vi "Ratchet Brake.vi"(4 "Untension Speed":dbl=-0.1, 5 "Slow Extend":dbl=0.25, 6 "Brake Delay":dbl=0.2, 7 "Extend Speed":dbl=1.0, 8 "Reverse Time":dbl=0.4, 9 "Slow Retract":dbl=-0.25, 10 "Servo Disengage":i32, 11 "Retract Speed":dbl=-0.9, 12 "Retract":bool, 13 "Extend":bool, 14 "Slow":bool, 15 "Servo Engage":i32=120) -> (1 "Motor":dbl, 2 "Brake Servo":i32, 3 "State":enum16{"Engaged", "Untension", "Disengaged"}(ring))   [LabVIEW 2012]
panel:
  in  "Retract 2":bool
  in  "Extend 2":bool
  in  "Slow 2":bool
  out "State 2":enum16{"Engaged", "Untension", "Disengaged"}(ring)
  # "INPUTS"
  # "BRAKE SETTINGS"
  # "OUTPUTS"
  # "Disabled Code Implementation Example"
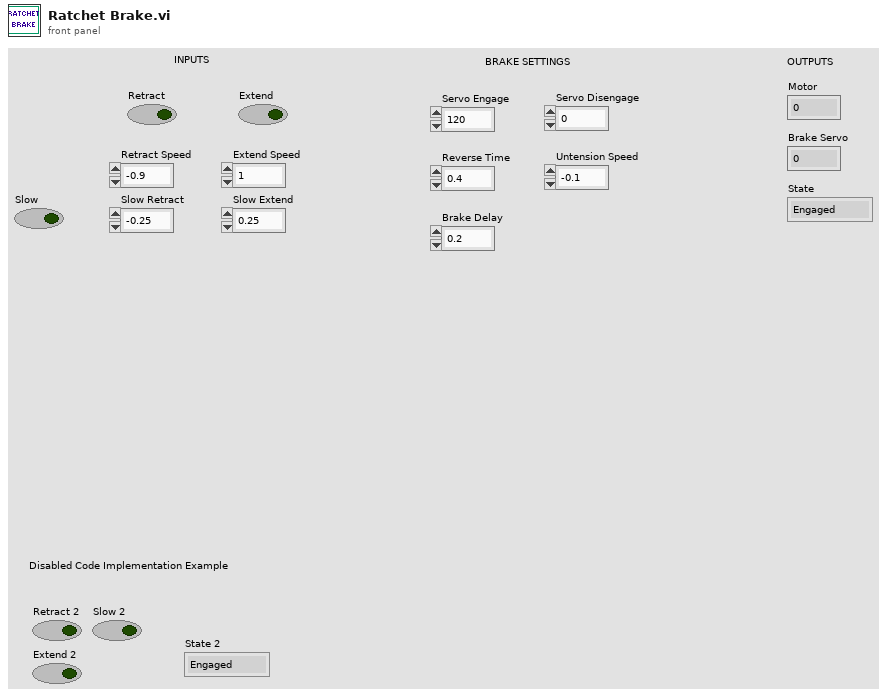
[diagram p1: front panel]
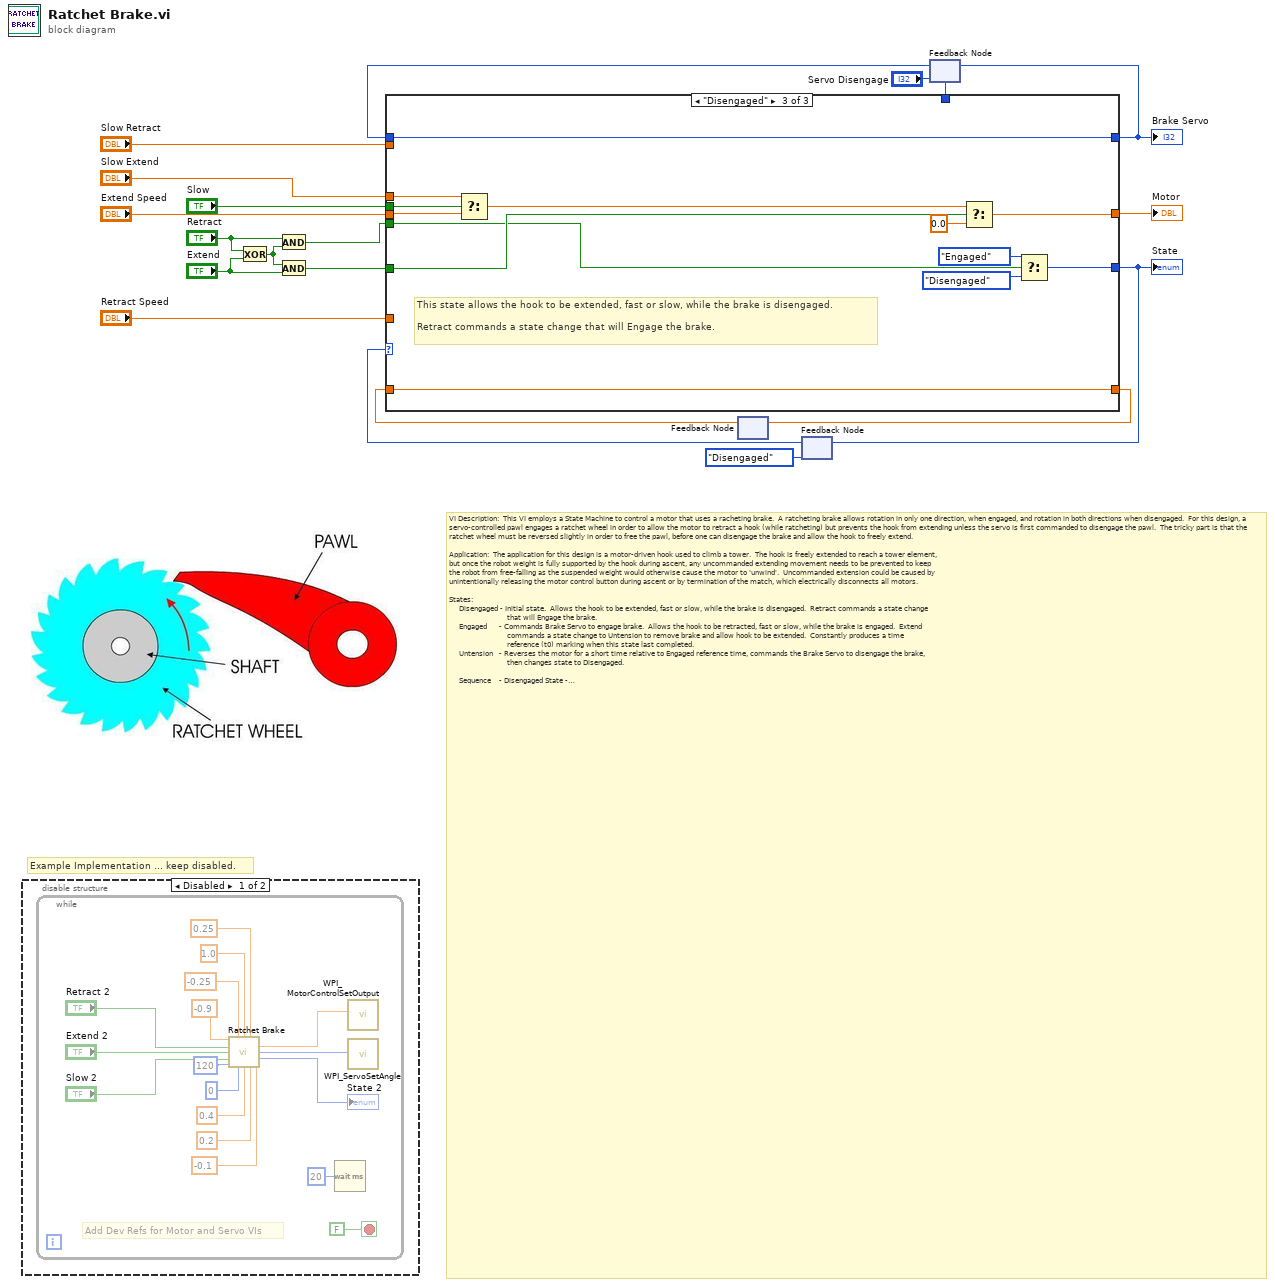
[diagram p0: block diagram]
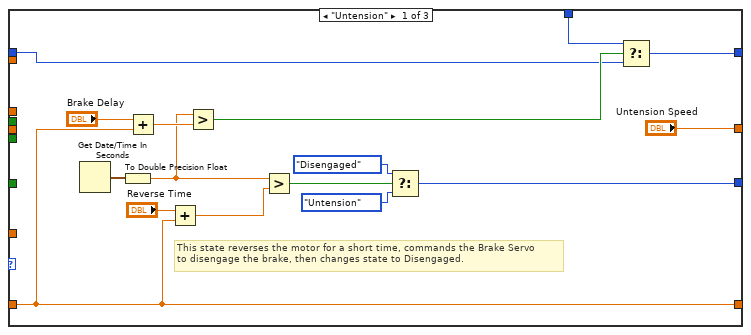
[diagram p3: hidden frame]
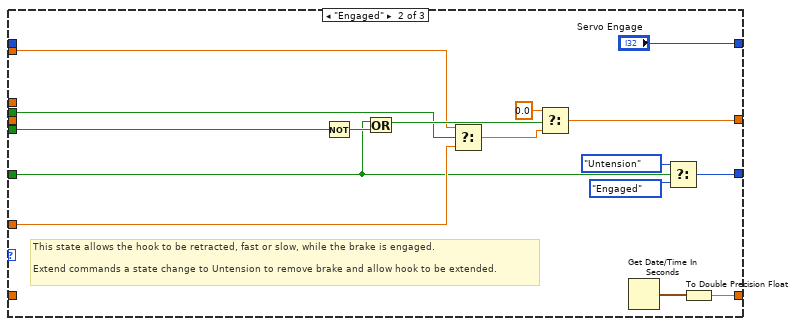
[diagram p4: hidden frame]
diagram:
  # "Example Implementation ... keep disabled."
  # "VI Description:  This VI employs a State Machine to control a motor that uses a racheting brake.  A ratcheting brake allows rotation in only one direction, when engaged, and rotation in both directions when disengaged.  For this design, a servo-controlled pawl engages a ratchet wheel in order to allow the motor to retract a hook (while ratcheting) but prevents the hook from extending unless the servo is first commanded to disengage the pawl.  The tricky part is that the ratchet wheel must be reversed slightly in order to free the pawl, before one can disengage the brake and allow the hook to freely extend.\n\nApplication:  The application for this design is a motor-driven hook used to climb a tower.  The hook is freely extended to reach a tower element,\nbut once the robot weight is fully supported by the hook during ascent, any uncommanded extending movement needs to be prevented to keep\nthe robot from free-falling as the suspended weight would otherwise cause the motor to 'unwind'.  Uncommanded extension could be caused by \nunintentionally releasing the motor control button during ascent or by termination of the match, which electrically disconnects all motors.\n\nStates:  \n     Disengaged - Initial state.  Allows the hook to be extended, fast or slow, while the brake is disengaged.  Retract commands a state change\n                             that will Engage the brake.\n     Engaged      - Commands Brake Servo to engage brake.  Allows the hook to be retracted, fast or slow, while the brake is engaged.  Extend \n                             commands a state change to Untension to remove brake and allow hook to be extended.  Constantly produces a time\n                             reference (t0) marking when this state last completed.\n     Untension   - Reverses the motor for a short time relative to Engaged reference time, commands the Brake Servo to disengage the brake,\n                             then changes state to Disengaged.\n\n     Sequence    - Disengaged State -> (on retract) -> Engaged State -> (on extend) -> Untension State -> Disengaged State\n\nThe state machine principle is that the brake is engaged whenever retracting (climbing).  The brake is untensioned by reversing the ratchet\nwheel upon an extend command.  This effectively allows extension to only occur when specifically commanded.\n\nInputs:\n     Extend                   - Boolean command to extend hook.  Simultaneous selection of Extend and Retract is considered ambigious and results in no change.\n     Retract                  - Boolean command to retract hook.  Simultaneous selection of Extend and Retract is considered ambigious and results in no change.\n     Slow                      - Use Slow Extend or Slow Retract motor values when True.\n     Extend Speed       - Motor value for fast extend.\n     Retract Speed      - Motor value for fast retract.\n     Slow Extend         - Motor value for slow extend.\n     Slow Retract         - Motor value for slow retract.\n     Untension Speed - Motor value to reverse motor while untensioning brake.\n     Reverse Time       - Time in seconds to reverse motor while untensioning brake.\n     Brake Delay          - Time in seconds to delay prior to commanding brake servo to remove brake pawl.\n     Servo Engage       - Servo position to move brake pawl into ratchet wheel.\n     Servo Disengage - Servo position to remove brake pawl from ratchet wheel.\n\nOutputs:\n     Brake Servo          - Current Brake Servo position.\n     Motor                   - Motor value output determined by state machine.\n     State                     - Current state of state machine.\n\nImplementation:\n     Determine Brake Servo positions for moving brake pawl into and out of ratchet wheel, and set Servo Engage and Disengage.\n     Determine a motor Untension Speed and Reverse Time combination that allows the brake pawl to be freed from the ratchet wheel at Brake\n           Delay seconds.  Reverse Time and Brake Delay will likely be fractions of a second, with Reverse Time >= Brake Delay.\n     Set Extend, Retract, and Slow speed motor values.  Extend and Retract will have opposite signs.  Untension Speed will have the same sign as Retract.\n\n\n----- RoboBees Team 836! -----  Control your freewheeling, think about a career in STEM! ..."
  n1 = disable-structure shown="Disabled" {
    frame Disabled {
      n2 = while {
        stop <- FALSE stop-if-true
        # "Add Dev Refs for Motor and Servo VIs"
        n3 = call "Ratchet Brake.vi"("Untension Speed"=-0.1, "Slow Extend"=0.25, "Brake Delay"=0.2, "Extend Speed"=1.0, "Reverse Time"=0.4, "Slow Retract"=-0.25, "Servo Disengage"=0, "Retract Speed"=-0.9, "Retract"="Retract 2", "Extend"="Extend 2", "Slow"="Slow 2", "Servo Engage"=120) -> ("Motor"=w21:dbl, "Brake Servo"=w20:i32, "State"=→"State 2":enum16{"Engaged", "Untension", "Disengaged"})  [unwired: 1 in]
        n4 = Wait (ms)(milliseconds to wait=u32 20) -> ()  [unwired: 1 out]
        n5 = call <vilib>:"WPI_MotorControlSetOutput.vi"("Output"=w21) -> ()  [unwired: 8 in, 3 out]
        n6 = call <vilib>:"WPI_ServoSetAngle.vi"("Angle"=w20) -> ()  [unwired: 9 in, 2 out]
      }
    }
    frame Enabled {
    }
  }
  n7 = Exclusive Or(1:"Extend", 2:"Retract") -> (0:w3:bool)
  n8 = And(x="Retract", y=w3) -> (x .and. y?=w2:bool)
  n9 = And(x=w3, y="Extend") -> (x .and. y?=w1:bool)
  n10 = feedback #1() -> (w17:dbl)  [unwired: 1 in]
  n11 = feedback #2(enum16{"Engaged", "Untension", "Disengaged"}."Disengaged") -> (w19:enum16{"Engaged", "Untension", "Disengaged"})
  n12 = feedback #3("Servo Disengage") -> (w7:i32)
  n13 = case shown="\"Disengaged\"" w19 {
    tunnel: [w50 w68 w81] -> w15
    tunnel: ["Untension Speed" w63 w78] -> w14
    tunnel: [w42 w61 w77] -> w18
    tunnel: w17 -> [w42 _ w77]
    tunnel: w1 -> [_ w54 w72]
    tunnel: w2 -> [_ w58 w70]
    tunnel: "Retract Speed" -> [_ w57 _]
    tunnel: "Slow" -> [_ w56 w73]
    tunnel: "Extend Speed" -> [_ _ w74]
    tunnel: "Slow Extend" -> [_ _ w71]
    tunnel: "Slow Retract" -> [_ w55 _]
    tunnel: [w40 "Servo Engage" w69] -> w8
    tunnel: w7 -> [w38 _ w69]
    tunnel: "Servo Disengage" -> [w37 _ _]
    frame "Untension" {
      # "This state reverses the motor for a short time, commands the Brake Servo\nto disengage the brake, then changes state to Disengaged."
      n14 = Get Date/Time In Seconds() -> (seconds since 1Jan1904=w52:timestamp)
      n15 = To Double Precision Float(number=w52) -> (double precision float=w43:dbl)
      n16 = Add(x="Brake Delay", y=w42) -> (x+y=w44:dbl)
      n17 = Add(x="Reverse Time", y=w42) -> (x+y=w49:dbl)
      n18 = Greater?(x=w43, y=w44) -> (0:w39:bool)
      n19 = Greater?(x=w43, y=w49) -> (0:w51:bool)
      n20 = Select(t=enum16{"Engaged", "Untension", "Disengaged"}."Disengaged", s=w51, f=enum16{"Engaged", "Untension", "Disengaged"}."Untension") -> (s? t:f=w50:enum16{"Engaged", "Untension", "Disengaged"})
      n21 = Select(t=w37, s=w39, f=w38) -> (s? t:f=w40:i32)
    }
    frame "Engaged" {
      # "This state allows the hook to be retracted, fast or slow, while the brake is engaged.\n\nExtend commands a state change to Untension to remove brake and allow hook to be extended."
      n22 = Not(x=w58) -> (.not. x?=w67:bool)
      n23 = Or(x=w54, y=w67) -> (x .or. y?=w65:bool)
      n24 = Select(t=w55, s=w56, f=w57) -> (s? t:f=w66:dbl)
      n25 = Select(t=0.0, s=w65, f=w66) -> (s? t:f=w63:dbl)
      n26 = Get Date/Time In Seconds() -> (seconds since 1Jan1904=w62:timestamp)
      n27 = Select(t=enum16{"Engaged", "Untension", "Disengaged"}."Untension", s=w54, f=enum16{"Engaged", "Untension", "Disengaged"}."Engaged") -> (s? t:f=w68:enum16{"Engaged", "Untension", "Disengaged"})
      n28 = To Double Precision Float(number=w62) -> (double precision float=w61:dbl)
    }
    frame "Disengaged" {
      # "This state allows the hook to be extended, fast or slow, while the brake is disengaged.\n\nRetract commands a state change that will Engage the brake."
      n29 = Select(t=w71, s=w73, f=w74) -> (s? t:f=w80:dbl)
      n30 = Select(t=w80, s=w72, f=0.0) -> (s? t:f=w78:dbl)
      n31 = Select(t=enum16{"Engaged", "Untension", "Disengaged"}."Engaged", s=w70, f=enum16{"Engaged", "Untension", "Disengaged"}."Disengaged") -> (s? t:f=w81:enum16{"Engaged", "Untension", "Disengaged"})
    }
  }
  "State" <- w15
  "Motor" <- w14
  "Brake Servo" <- w8
  n32 = feedback-in #1(w18) -> ()
  n33 = feedback-in #2(w15) -> ()
  n34 = feedback-in #3(w8) -> ()
